vi "Binary to Images.vi"() -> ()   [LabVIEW 2013]
panel:
  in  "stop":bool
  out "Progress":u64(slide) max=5098 scale=0.0..5098.0
  out "Partial images in file?":bool
  out "# of Images":u32
  out "error IO":errorcluster
  out "Height":u32
  out "Width":u32
  out "size (in bytes)":i64
  in  "Created Image Path":path
  in  "Binary File":path
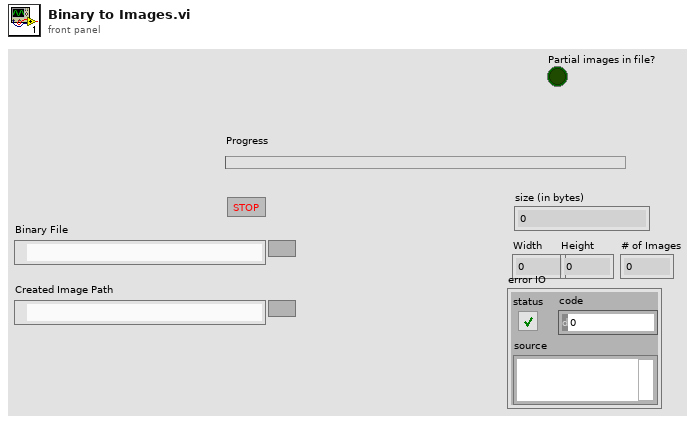
[diagram p1: front panel]
types:
  T1 = typedef "Image Type" = u32
  T2 = enum16{"open", "replace", "create", "open or create", "replace or create", "replace or create with confirmation"}
  T3 = typedef "IMAQ Image.ctl" = refnum<image>
  T4 = enum16{"big-endian, network order", "native, host order", "little-endian"}
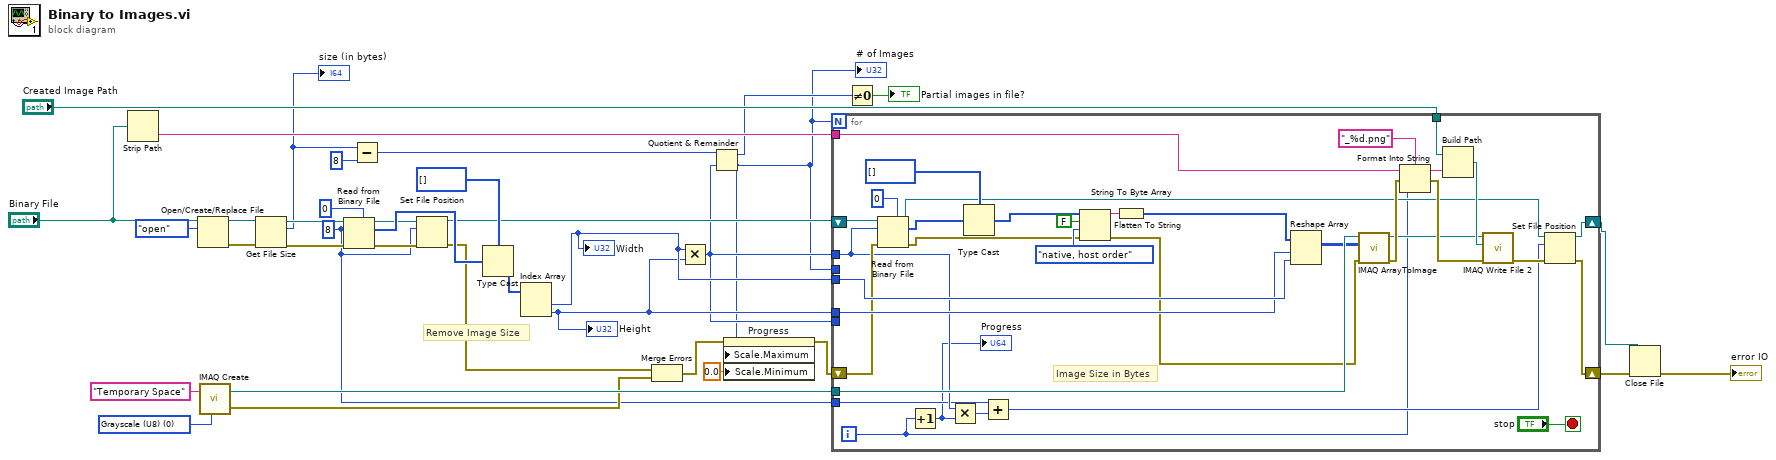
[diagram p0: block diagram]
diagram:
  w5 = 8 ("count (1)")
  w29 = T1 0 items=["Grayscale (U8)", "Grayscale (I16)", "Grayscale (SGL)", "Complex (CSG)", "RGB (U32)", "HSL (U32)", "RGB (U64)", "Grayscale (U16)"] ("Image Type")
  # "Remove Image Size"
  n1 = Strip Path(path="Binary File") -> (name=w24:string)  [unwired: 1 out]
  n2 = Open/Create/Replace File(file path (use dialog)="Binary File", operation (0:open)=T2."open") -> (refnum out=w35:refnum<file>, error out=w34:errorcluster)  [unwired: 4 in, 1 out]
  n3 = call "IMAQ Create"("Image Name"="Temporary Space", "Image Type"=w29) -> ("New Image"=w28:T3, "error out"=w27:errorcluster)  [unwired: 3 in]
  n4 = Get File Size(file=w35, error in=w34) -> (refnum out=w32:refnum<file>, size (in bytes)=w18:i64, 0:w33:errorcluster)
  "size (in bytes)" <- w18
  n5 = Read from Binary File(5:u8 0, 8:w33, 10:w5, 11:w32) -> (0:w10:errorcluster, 2:w31:u8[], 3:w11:refnum<file>)  [unwired: 2 in, 1 out]
  n6 = Subtract(x=w18, y=i64 8) -> (x-y=w16:i64)
  n7 = Set File Position(offset (in bytes) (0)=w5, refnum=w11, error in=w10) -> (refnum out=w8:refnum<file>, error out=w9:errorcluster)  [unwired: 1 in]
  n8 = Type Cast(type=u32[] [], x=w31) -> (*(type *) &x=w21:u32[])
  n9 = Index Array(array=w21) -> (element #1=w20:u32, element #2=w19:u32)  [unwired: 2 in]
  "Width" <- w20
  "Height" <- w19
  n10 = Merge Errors(w9, w27) -> (w4:errorcluster)
  n11 = Multiply(x=w20, y=w19) -> (x*y=w7:u32)
  n12 = Quotient & Remainder(x=w16, y=w7) -> (x-y*floor(x/y)=w12:i64, floor(x/y)=w1:i64)
  "# of Images" <- w1
  n13 = property on="Progress" class="Slide (strict)"(error in=w4, "Scale.Maximum"=w1, "Scale.Minimum"=0.0 ("Data Entry Limits:Minimum")) -> (error out=w3:errorcluster)  [unwired: 1 in, 1 out]
  n14 = for {
    N: w1 -> [_]
    tunnel: w28 -> [w71]
    tunnel: "Created Image Path" -> [w70]
    tunnel: w24 -> [w69]
    tunnel: w20 -> [w68]
    tunnel: w19 -> [w67]
    tunnel: w7 -> [_]
    shift-right: [w43] -> w14
    shift-left: w3 -> [w53]
    shift-right: [w41] -> w6
    shift-left: w8 -> [w54]
    tunnel: w7 -> [w47]
    tunnel: w5 -> [w45]
    tunnel: w1 -> [_]
    i -> [w38]
    stop <- "stop" stop-if-true
    # "Image Size in Bytes"
    n15 = Read from Binary File(5:u8 0, 8:w53, 10:w47, 11:w54) -> (0:w52:errorcluster, 2:w50:u8[], 3:w42:refnum<file>)  [unwired: 2 in, 1 out]
    n16 = Increment(x=w38) -> (x+1=w37:i32)
    "Progress" <- w37
    n17 = Multiply(x=w47, y=w37) -> (x*y=w46:u32)
    n18 = Type Cast(type=u64[] [], x=w50) -> (*(type *) &x=w48:u64[])
    n19 = Add(x=w45, y=w46) -> (x+y=w40:u32)
    n20 = Flatten To String(anything=w48, prepend array or string size? (T)=FALSE, byte order (0:big-endian, network order)=T4."native, host order", error in (no error)=w52) -> (data string=w64:string, error out=w62:errorcluster)  [unwired: 1 out]
    n21 = String To Byte Array(string=w64) -> (unsigned byte array=w63:u8[])
    n22 = Reshape Array(w63, w67, w68) -> (w61:u8[][])
    n23 = call "IMAQ ArrayToImage"("error in (no error)"=w62, "Image Pixels (U8)"=w61, "Image"=w71) -> ("error out"=w58:errorcluster, "Image Out"=w55:T3)  [unwired: 7 in]
    n24 = Format Into String(format string="_%d.png", initial string=w69, error in=w58, w38) -> (resulting string=w59:string, error out=w57:errorcluster)
    n25 = Build Path(base path=w70, name or relative path=w59) -> (appended path=w56:path)
    n26 = call-poly "IMAQ Write File 2"("error in (no error)"=w57, "File Path"=w56, "Image"=w55) -> ("error out"=w44:errorcluster)  [unwired: 7 in, 1 out]
    n27 = Set File Position(offset (in bytes) (0)=w40, refnum=w42, error in=w44) -> (refnum out=w41:refnum<file>, error out=w43:errorcluster)  [unwired: 1 in]
  }
  n28 = Not Equal To 0?(x=w12) -> (x != 0?=→"Partial images in file?":bool)
  n29 = Close File(refnum=w6, error in=w14) -> (error out=→"error IO":errorcluster)  [unwired: 1 out]
